vi "ControlSystem.vi"() -> ()   [LabVIEW 2025]
uses:
  <vilib>/OPCUA/controls/NodeId.ctl
  <vilib>/OPCUA/controls/Write Status.ctl
  <vilib>/OPCUA/client/Connect2.vi
  <vilib>/OPCUA/client/Multiple Write Double.vi
  <vilib>/OPCUA/NI OPC UA Client.lvlib
  <vilib>/gmath/NI_Gmath.lvlib
panel:
  out "yk":dbl
  out "Control signal":dbl
  in  "Ts":dbl
  in  "Ti":dbl
  in  "Kp":dbl
  in  "rk":dbl
  in  "item node ID":T1
  in  "server endpoint URL":string
  in  "Log data":bool
  out "Air Heater Data":dbl[](graph)
  in  "?":bool
  out "Temperature [C]":dbl format="%#.1g"
  # "PI Controller"
  # "Air Heater Control System"
  # "OPC UA Server"
  # "Program Settings"
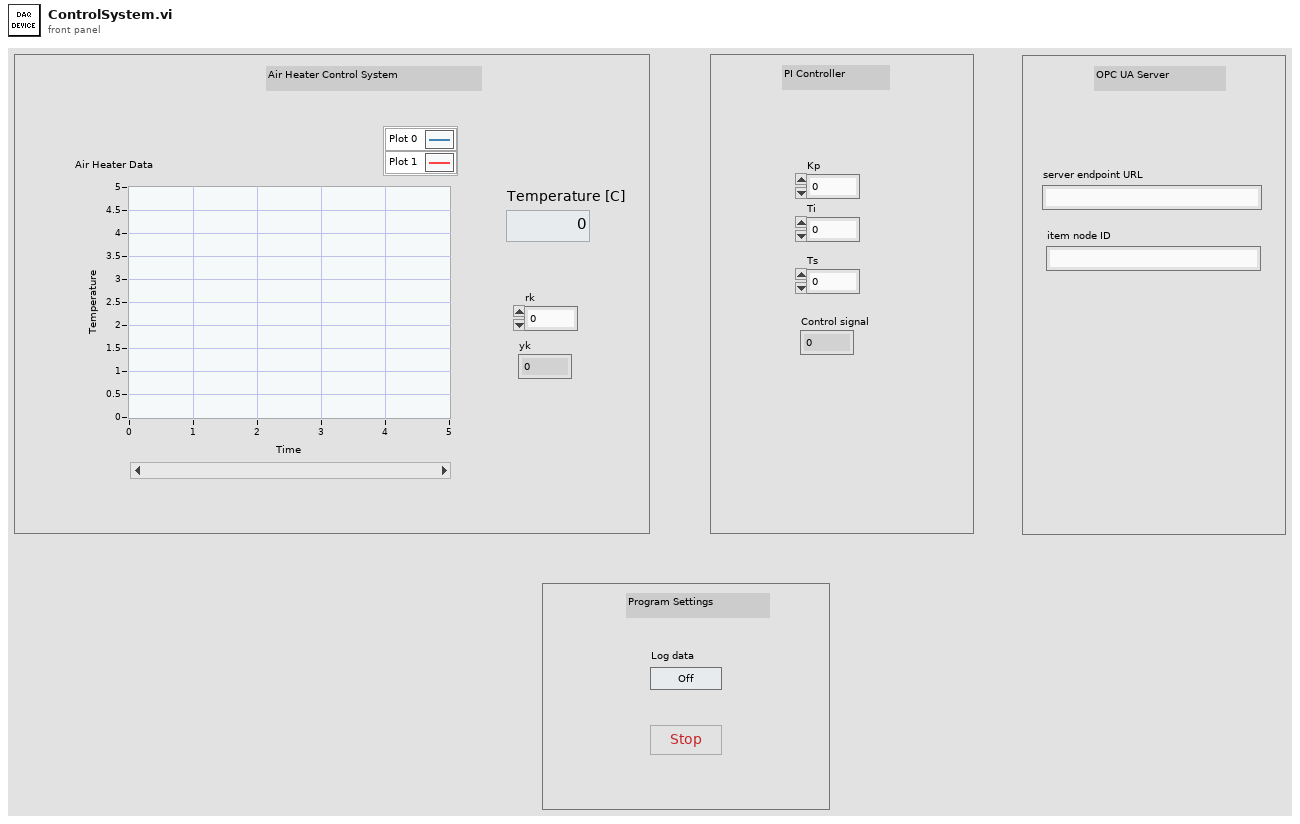
[diagram p1: front panel]
types:
  T1 = typedef "NodeId.ctl" = string
  T2 = typedef "OPC UA Client Refnum.ctl" = refnum<k21>
  T3 = typedef "Write Status.ctl" = u32
  T4 = cluster{"node ID":T1, "value":dbl, "timestamp (current time)":timestamp, "node status":T3}
  T5 = cluster{"node ID":T1, "value":dbl, "timestamp (current time)":timestamp, "node status":T3}[]
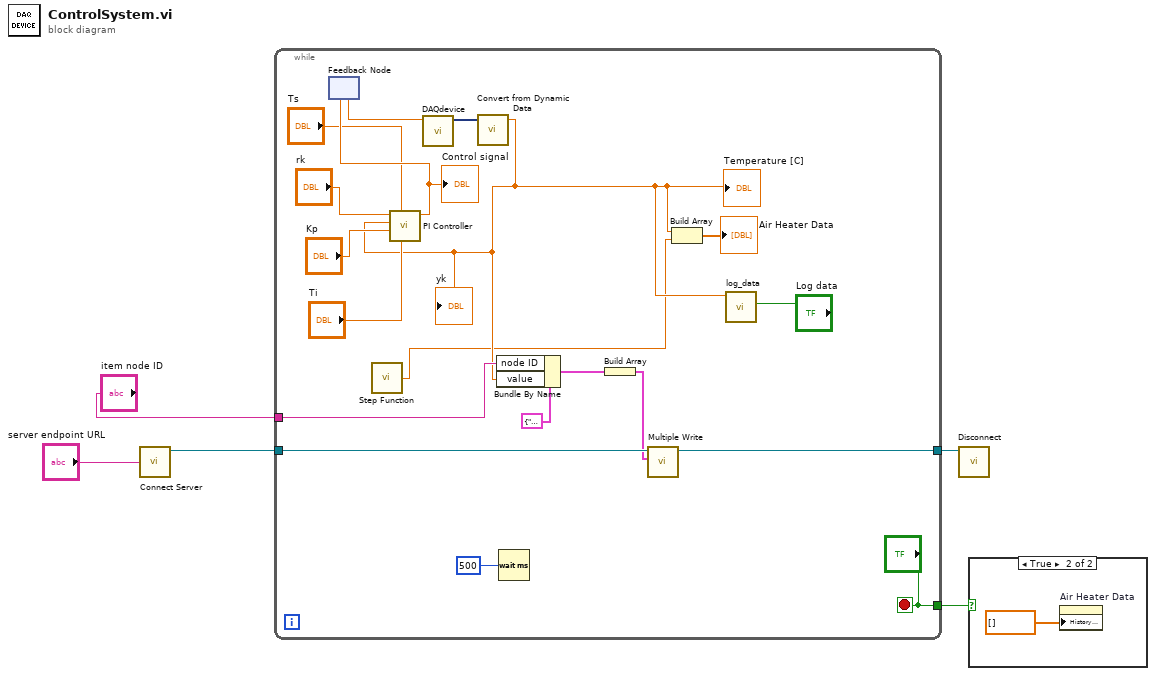
[diagram p0: block diagram]
diagram:
  n1 = call-poly <vilib>:"Connect Server.vi"("server endpoint URL"="server endpoint URL") -> ("OPC UA client refnum out"=w3:T2)  [unwired: 8 in, 2 out]
  n2 = while {
    tunnel: ["?"] -> w5
    tunnel: [w21] -> w4
    tunnel: w3 -> [w20]
    tunnel: "item node ID" -> [w16]
    stop <- "?" stop-if-true
    n3 = feedback #1() -> (w13:dbl)  [unwired: 1 in]
    n4 = call <vilib>:"Step Function.vi"() -> ("step(x)"=w8:dbl)  [unwired: 1 in]
    n5 = call "DAQdevice.vi"("data in"=w13) -> ("data out"=w15:dynamicdata)  [unwired: 10 in]
    n6 = call "Convert from Dynamic Data"("Dynamic Data Type"=w15) -> ("Scalar"=w9:dbl)  [unwired: 3 in]
    "Temperature [C]" <- w9
    "yk" <- w9
    n7 = call "PI Controller.vi"("Ti"="Ti", "Ts"="Ts", "Kp"="Kp", "yk"=w9, "rk"="rk") -> ("Control signal"=w14:dbl)  [unwired: 6 in]
    "Control signal" <- w14
    n8 = feedback-in #1(w14) -> ()
    n9 = Bundle By Name "Bundle By Name"(cluster=T4 {"node ID"="", "value"=0.0, "timestamp (current time)"=timestamp(0 s since 1904-01-01), "node status"=0} ("request"), "node ID"=w16, "value"=w9) -> (w19:T4)
    n10 = Wait (ms)(milliseconds to wait=u32 500 ("millisecond timer value")) -> ()  [unwired: 1 out]
    n11 = Build Array "Build Array"(w19) -> (w17:T5)
    n12 = call-poly <vilib>:"Multiple Write.vi"("requests"=w17, "OPC UA client refnum in"=w20) -> ("OPC UA client refnum out"=w21:T2)  [unwired: 6 in, 3 out]
    n13 = Build Array(w9, w8) -> (→"Air Heater Data":dbl[])
    n14 = call "log_data.vi"("Log data"="Log data", "data"=w9) -> ()  [unwired: 10 in]
  }
  n15 = call <vilib>:"Disconnect.vi"("OPC UA client refnum in"=w4) -> ()  [unwired: 10 in, 1 out]
  n16 = case shown="True" w5 {
    frame False {
    }
    frame True {
      n17 = property on="Air Heater Data" class="WFChart (strict)"("History Data"=dbl[] []) -> ()  [unwired: 2 in, 2 out]
    }
  }
